vi "Example-AnalogInSimple.vi"() -> ()   [LabVIEW 2018]
panel:
  out "Scope Graph":cluster{"voltages":dbl[], "voltages":dbl[]}[](graph) caption="XY图"
  in  "trigcond":enum16{"Raising", "Falling", "Either"}(ring)
  in  "trigsrc":T1(ring)
  in  "trigtype":enum16{"edge", "pulse", "trasition"}(ring)
  in  "range 2":dbl=5.0
  in  "voltsLevel":dbl
  in  "timeout":i32
  in  "range":dbl=5.0
  in  "buffersize":i32=2048
  out "returns":i32[](array[numeric])
  in  "fre":i32=800000
  out "error out":errorcluster caption="错误输出"
  in  "error in (no error)":errorcluster caption="错误输入（无错误）"
  out "ftHandle out":u64=363562184
  in  "设备索引":i32
  # "0x0FFF"
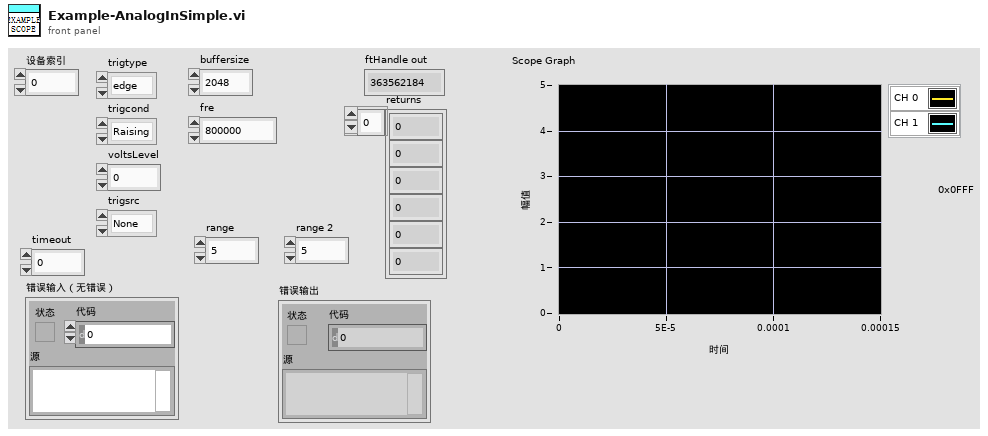
[diagram p1: front panel]
types:
  T1 = enum16{"None", "DetectorAnalogInCH1", "DetectorAnalogInCH2", "AnalogOut1", "AnalogOut2", "DetectorDigitalIn", "DigitalOut", "Manule", "External 1", "External 2", "DigitalIn"}
  T2 = enum16{"CLIFFStateReady", "CLIFFStateArmed", "CLIFFStateDone", "CLIFFStateRunning", "CLIFFStateConfig", "CLIFFStatePrefill", "CLIFFStateTriggered", "CLIFFStateWait"}
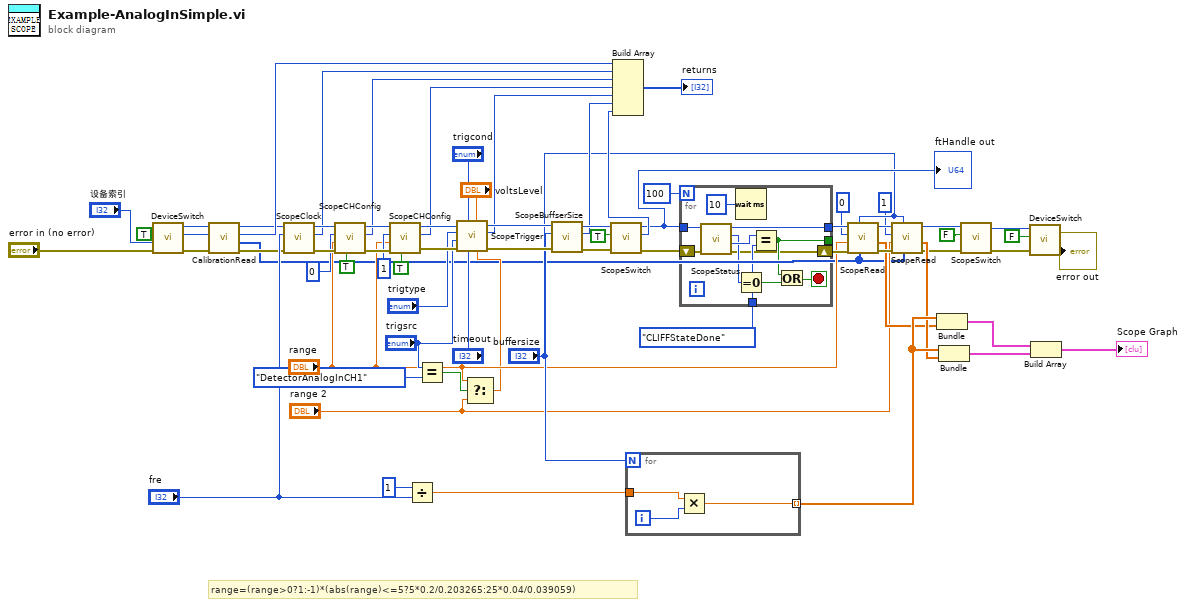
[diagram p0: block diagram]
diagram:
  # "range=(range>0?1:-1)*(abs(range)<=5?5*0.2/0.203265:25*0.04/0.039059)"
  n1 = call "DeviceSwitch.vi"("error in (no error)"="error in (no error)", "Device Index"="设备索引", "Open"=TRUE) -> ("error out"=w2:errorcluster, "function return"=w37:i32, "handle out"=w5:u64)  [unwired: 4 in, 2 out]
  n2 = call "CalibrationRead.vi"("handle"=w5, "error in (no error)"=w2) -> ("handle out"=w4:u64, "CalArray"=w1:u8[], "error out"=w3:errorcluster)  [unwired: 5 in, 1 out]
  n3 = call "ScopeClock.vi"("error in (no error)"=w3, "fre(Hz)"="fre", "handle"=w4) -> ("error out"=w49:errorcluster, "function return"=w36:i32, "handle out"=w58:u64)  [unwired: 6 in]
  n4 = call "ScopeCHConfig.vi"("enable"=TRUE, "error in (no error)"=w49, "range(V)"="range", "CH"=0 ("channel 3"), "handle"=w58) -> ("error out"=w48:errorcluster, "function return"=w35:i32, "handle out"=w59:u64)  [unwired: 4 in]
  n5 = call "ScopeCHConfig.vi"("enable"=TRUE, "error in (no error)"=w48, "range(V)"="range", "CH"=1 ("channel 2"), "handle"=w59) -> ("error out"=w56:errorcluster, "function return"=w34:i32, "handle out"=w57:u64)  [unwired: 4 in]
  n6 = Divide(x=1, y="fre") -> (x/y=w64:dbl)
  n7 = Equal?(x="trigsrc", y=T1."DetectorAnalogInCH1") -> (x = y?=w9:bool)
  n8 = Select(t="range", s=w9, f="range 2") -> (s? t:f=w6:dbl)
  n9 = call "ScopeTrigger.vi"("range"=w6, "voltsLevel"="voltsLevel", "timeout"="timeout", "trigcond"="trigcond", "error in (no error)"=w56, "trigsrc"="trigsrc", "trigtype"="trigtype", "handle"=w57) -> ("error out"=w55:errorcluster, "function return"=w33:i32, "handle out"=w54:u64)  [unwired: 1 in]
  n10 = call "ScopeBuffserSize.vi"("error in (no error)"=w55, "BufferSize"="buffersize", "handle"=w54) -> ("error out"=w47:errorcluster, "function return"=w32:i32, "handle out"=w53:u64)  [unwired: 6 in]
  n11 = call "ScopeSwitch.vi"("error in (no error)"=w47, "Run"=TRUE ("run"), "handle"=w53) -> ("error out"=w38:errorcluster, "function return"=w31:i32, "handle out"=w30:u64)  [unwired: 6 in]
  "ftHandle out" <- w30
  n12 = Build Array(w37, w36, w35, w34, w33, w32, w31) -> (→"returns":i32[])
  n13 = for {
    N: "buffersize" -> [_]
    tunnel: w64 -> [w70]
    tunnel: [w69] -> w60 mode=indexing
    i -> [w71]
    n14 = Multiply(x=w70, y=w71) -> (x*y=w69:dbl)
  }
  n15 = for {
    N: 100 -> [_]
    tunnel: w30 -> [w76]
    shift-right: [w72] -> w23
    shift-left: w38 -> [w77]
    tunnel: T2."CLIFFStateDone" ("ANIStatus") -> [w82]
    tunnel: [w75] -> w24
    tunnel: [w81] -> _
    stop <- w79 stop-if-true
    n16 = call "ScopeStatus.vi"("error in (no error)"=w77, "handle"=w76) -> ("error out"=w72:errorcluster, "ANIStatus"=w74:T2, "function return"=w73:i32, "handle out"=w75:u64)  [unwired: 6 in]
    n17 = Wait (ms)(milliseconds to wait=u32 10 ("等待时间（毫秒）")) -> ()  [unwired: 1 out]
    n18 = Equal To 0?(x=w73) -> (x = 0?=w78:bool)
    n19 = Equal?(x=w74, y=w82) -> (x = y?=w81:bool)
    n20 = Or(x=w81, y=w78) -> (x .or. y?=w79:bool)
  }
  n21 = call "ScopeRead.vi"("CalArray"=w1, "BufferSize"="buffersize", "error in (no error)"=w23, "Range"="range", "ch"=0, "handle"=w24) -> ("error out"=w26:errorcluster, "voltages"=w19:dbl[], "handle out"=w25:u64)  [unwired: 1 in, 2 out]
  n22 = call "ScopeRead.vi"("CalArray"=w1, "BufferSize"="buffersize", "error in (no error)"=w26, "Range"="range 2", "ch"=1, "handle"=w25) -> ("error out"=w12:errorcluster, "voltages"=w20:dbl[], "handle out"=w13:u64)  [unwired: 1 in, 2 out]
  n23 = Bundle(w60, "voltages"=w19) -> (w63:cluster{dbl[], "voltages":dbl[]})  [unwired: 1 in]
  n24 = Bundle(w60, "voltages"=w20) -> (w62:cluster{dbl[], "voltages":dbl[]})  [unwired: 1 in]
  n25 = call "ScopeSwitch.vi"("error in (no error)"=w12, "Run"=FALSE, "handle"=w13) -> ("error out"=w15:errorcluster, "handle out"=w14:u64)  [unwired: 6 in, 1 out]
  n26 = call "DeviceSwitch.vi"("error in (no error)"=w15, "Open"=FALSE, "handle"=w14) -> ("error out"=→"error out":errorcluster)  [unwired: 4 in, 4 out]
  n27 = Build Array(w63, w62) -> (→"Scope Graph":cluster{dbl[], "voltages":dbl[]}[])
